vi "Start Discovery Service.vi"(8 "error in":errorcluster, 11 "key file path":path) -> (0 "error out":errorcluster)   [LabVIEW 2020, in "MeasurementLink Measurement Server.lvlib"]
doc: "This VI starts the MeasurementLink.DiscoveryService.exe."
uses:
  MeasurementLink Measurement Server.lvlib
  <vilib>/Utility/sysdir.llb/System Directory Type.ctl
  Error Strings Global.vi
  <vilib>/ErrorRing/Error Ring.xnode
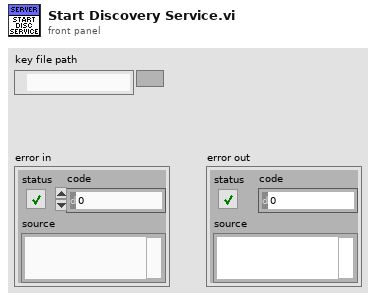
[diagram p1: front panel]
types:
  T1 = enum16{"open", "replace", "create", "open or create", "replace or create", "replace or create with confirmation"}
  T2 = typedef "System Directory Type.ctl" = i32
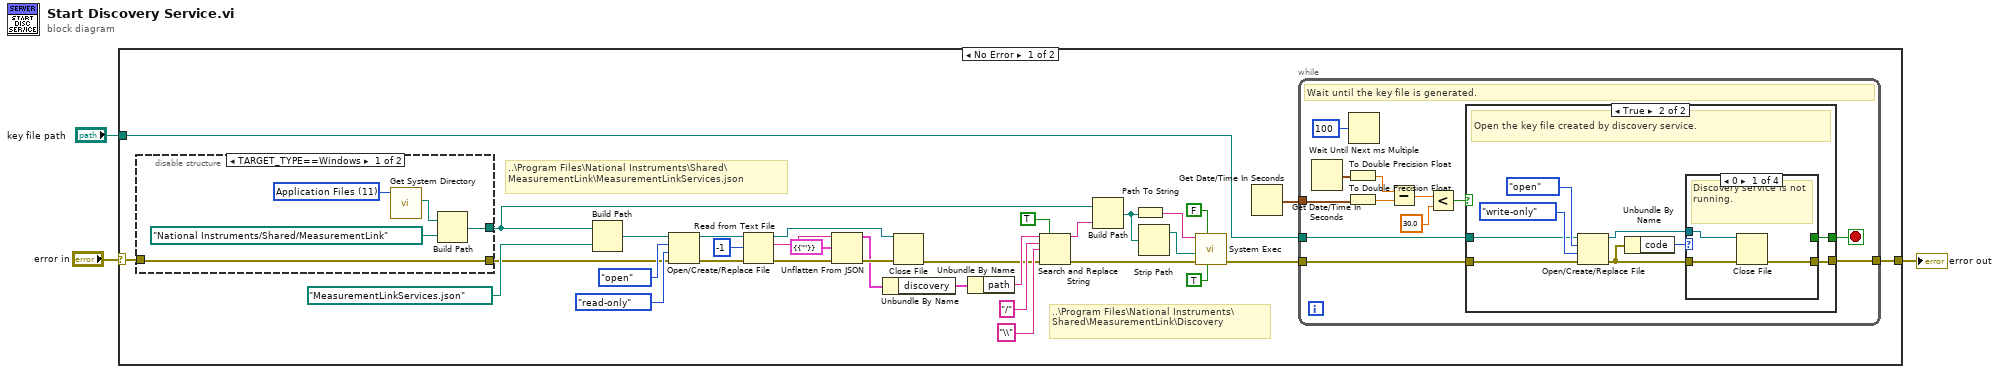
[diagram p0: block diagram]
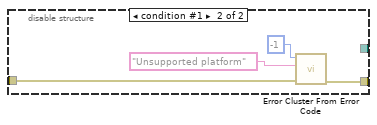
[diagram p2: hidden frame]
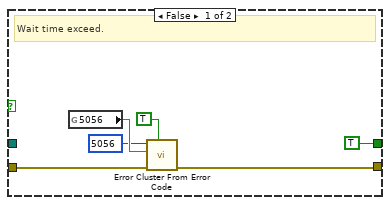
[diagram p3: hidden frame]
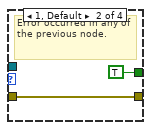
[diagram p4: hidden frame]
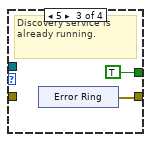
[diagram p5: hidden frame]
diagram:
  n1 = case shown="No Error" "error in" {
    selector: "error in" -> [w6 w82]
    tunnel: [w5 w82] -> w2
    tunnel: "key file path" -> [w4 _]
    frame No Error {
      # "..\\Program Files\\National Instruments\\Shared\\MeasurementLink\\Discovery"
      # "..\\Program Files\\National Instruments\\Shared\\MeasurementLink\\MeasurementLinkServices.json"
      n2 = disable-structure shown="TARGET_TYPE==Windows" {
        disable-tunnel: [w38 _] -> w8
        disable-tunnel: w6 -> [w37 w43]
        disable-tunnel: [w37 w42] -> w7
        frame condition #0 (active) {
          w41 = T2 11 items=["User Home"=0, "User Desktop"=1, "User Documents"=2, "User Application Data"=3, "User Preferences"=4, "User Temporary"=5, "Public Documents"=6, "Public Application Data"=7, "Public Preferences"=8, "Public Cache"=13, "System Core Libraries"=9, "System Installed Libraries"=10, "Application Files"=11, "Boot Volume Root"=12] ("system directory type")
          n3 = call <vilib>:"Get System Directory.vi"("system directory type"=w41) -> ("system directory"=w40:path)  [unwired: 10 in]
          n4 = Build Path(base path=w40, name or relative path=path "National Instruments/Shared/MeasurementLink") -> (appended path=w38:path)
        }
        frame condition #1 {
          n5 = call <vilib>:"Error Cluster From Error Code.vi"("error in (no error)"=w43, "error message (\"\")"="Unsupported platform" ("error message (\"\")"), "error code (0)"=-1) -> ("error out"=w42:errorcluster)  [unwired: 6 in]
        }
      }
      n6 = Build Path(base path=w8, name or relative path=path "MeasurementLinkServices.json") -> (appended path=w35:path)
      n7 = Open/Create/Replace File(file path (use dialog)=w35, error in=w7, operation (0:open)=T1."open", access (0:read/write)=enum16{"read/write", "read-only", "write-only"}."read-only") -> (refnum out=w32:refnum<file>, error out=w30:errorcluster)  [unwired: 2 in, 1 out]
      n8 = Read from Text File(file (use dialog)=w32, count=-1, error in=w30) -> (refnum out=w29:refnum<file>, text=w28:string, error out=w26:errorcluster)  [unwired: 1 in, 1 out]
      n9 = Unflatten From JSON(JSON string=w28, type and defaults=cluster{"discovery":cluster{"path":string}} {"discovery"={"path"=""}}, error in (no error)=w26) -> (value=w24:cluster{"discovery":cluster{"path":string}}, error out=w25:errorcluster)  [unwired: 4 in]
      n10 = Unbundle By Name(w24) -> ("discovery"=w23:cluster{"path":string})
      n11 = Close File(refnum=w29, error in=w25) -> (error out=w19:errorcluster)  [unwired: 1 out]
      n12 = Unbundle By Name(w23) -> ("path"=w22:string)
      n13 = Search and Replace String(replace all?=TRUE ("replace all? (F)"), input string=w22, search string="/", replace string="\\" ("replace string (\"\")"), error in=w19) -> (result string=w18:string, error out=w14:errorcluster)  [unwired: 3 in, 2 out]
      n14 = Build Path(base path=w8, name or relative path=w18) -> (appended path=w17:path)
      n15 = Path To String(path=w17) -> (string=w15:string)
      n16 = Strip Path(path=w17) -> (stripped path=w16:path)  [unwired: 1 out]
      n17 = call <vilib>:"System Exec.vi"("run minimized? (F)"=TRUE, "wait until completion? (T)"=FALSE, "error in (no error)"=w14, "working directory"=w16, "command line"=w15) -> ("error out"=w10:errorcluster)  [unwired: 3 in, 3 out]
      n18 = Get Date/Time In Seconds() -> (seconds since 1Jan1904=w11:timestamp)
      n19 = while {
        tunnel: w10 -> [w54]
        tunnel: w4 -> [w55]
        tunnel: [w52] -> w5
        tunnel: w11 -> [w47]
        stop <- w53 stop-if-true
        # "Wait until the key file is generated."
        n20 = Get Date/Time In Seconds() -> (seconds since 1Jan1904=w48:timestamp)
        n21 = To Double Precision Float(number=w48) -> (double precision float=w49:dbl)
        n22 = To Double Precision Float(number=w47) -> (double precision float=w46:dbl)
        n23 = Wait Until Next ms Multiple(millisecond multiple=u32 100) -> ()  [unwired: 1 out]
        n24 = Subtract(x=w49, y=w46) -> (x-y=w50:dbl)
        n25 = Less?(x=w50, y=30.0) -> (x < y?=w57:bool)
        n26 = case shown="True" w57 {
          tunnel: w55 -> [_ w69]
          tunnel: w54 -> [w59 w70]
          tunnel: [TRUE w65] -> w53
          tunnel: [w58 w66] -> w52
          frame False {
            # "Wait time exceed."
            n27 = global read "Error Strings Global.vi" "5056"() -> (w62:string)
            n28 = call <vilib>:"Error Cluster From Error Code.vi"("show call chain? (False)"=TRUE, "error in (no error)"=w59, "error message (\"\")"=w62, "error code (0)"=5056) -> ("error out"=w58:errorcluster)  [unwired: 5 in]
          }
          frame True {
            # "Open the key file created by discovery service."
            n29 = Open/Create/Replace File(file path (use dialog)=w69, error in=w70, operation (0:open)=T1."open", access (0:read/write)=enum16{"read/write", "read-only", "write-only"}."write-only") -> (refnum out=w64:refnum<file>, error out=w67:errorcluster)  [unwired: 2 in, 1 out]
            n30 = Unbundle By Name(w67) -> ("code"=w68:i32)
            n31 = case shown="0" w68 {
              tunnel: [w74 w77 w79 w81] -> w66
              tunnel: w67 -> [w75 w77 _ w81]
              tunnel: [_ TRUE TRUE _] -> w65
              tunnel: w64 -> [w73 _ _ _]
              frame 0 {
                # "Discovery service is not running."
                n32 = Close File(refnum=w73, error in=w75) -> (error out=w74:errorcluster)  [unwired: 1 out]
              }
              frame 1, Default {
                # "Error occurred in any of the previous node."
              }
              frame 5 {
                # "Discovery service is already running."
                n33 = xnode "Error Ring"() -> ("error out"=w79:errorcluster)
              }
              frame 7 {
                # "Key file is not created yet."
              }
            }
          }
        }
      }
    }
    frame Error {
    }
  }
  "error out" <- w2
